vi "Date formate.vi"() -> (3 "date string 2":string)   [LabVIEW 2017]
panel:
  out "time string":string
  out "date string":string
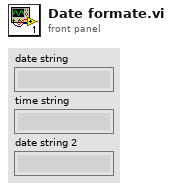
[diagram p1: front panel]
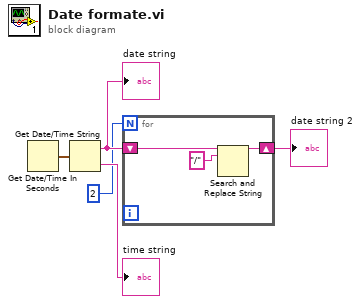
[diagram p0: block diagram]
diagram:
  n1 = Get Date/Time In Seconds() -> (seconds since 1Jan1904=w5:timestamp)
  n2 = Get Date/Time String(seconds (now)=w5) -> (date string=w3:string, time string=→"time string":string)  [unwired: 2 in]
  "date string" <- w3
  n3 = for {
    N: 2 -> [_]
    shift-right: [w6] -> w1
    shift-left: w3 -> [w8]
    n4 = Search and Replace String(input string=w8, search string="/") -> (result string=w6:string)  [unwired: 6 in, 3 out]
  }
  "date string 2" <- w1
